vi "read_stimulus_h5.vi"(11 "Path":path) -> (0 "error out":errorcluster, 3 "output cluster":T1, 4 "alignment_command":i32[](array[numeric]), 6 "piezo_command":i32[](array[numeric]))   [LabVIEW 2015]
uses:
  <vilib>/addons/h5labview2/file/H5Fmode.ctl
  <vilib>/addons/h5labview2/base/lib_path.vi
  <vilib>/addons/h5labview2/base/H5Equery.vi
  <vilib>/addons/h5labview2/base/hid_t.ctl
  <vilib>/addons/h5labview2/dataset/H5Dread.llb/H5Dread.xnode
  <vilib>/addons/h5labview2/file/H5F.lvlib
  <vilib>/addons/h5labview2/group/H5G.lvlib
panel:
  out "Alignment Command":dbl[](graph)
  out "Piezo Command":dbl[](graph)
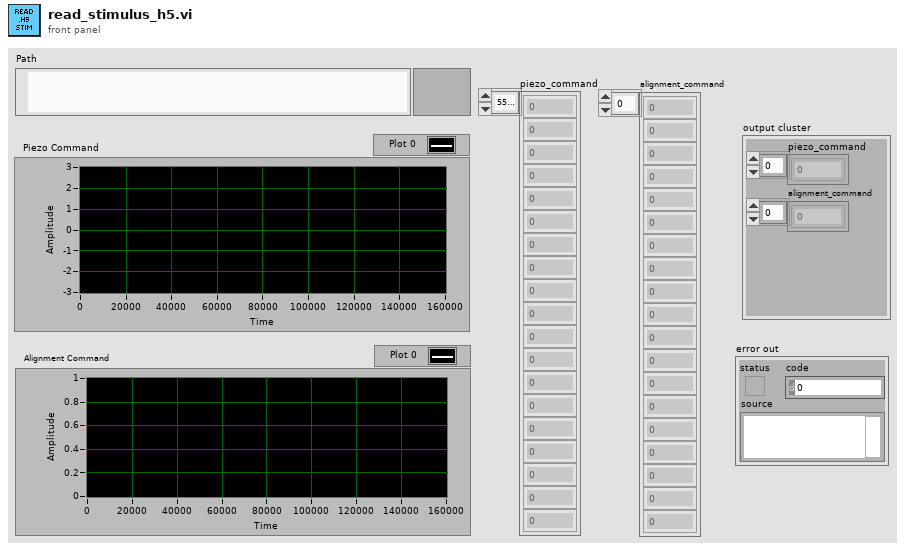
[diagram p1: front panel]
types:
  T1 = cluster{"piezo_command":dbl[], "alignment_command":dbl[]}
  T2 = typedef "H5F.lvlib/H5Fmode.ctl" = enum16{"read-only", "read-write", "overwrite", "create new", "open or create"}
  T3 = typedef "hid_t.ctl" = i32
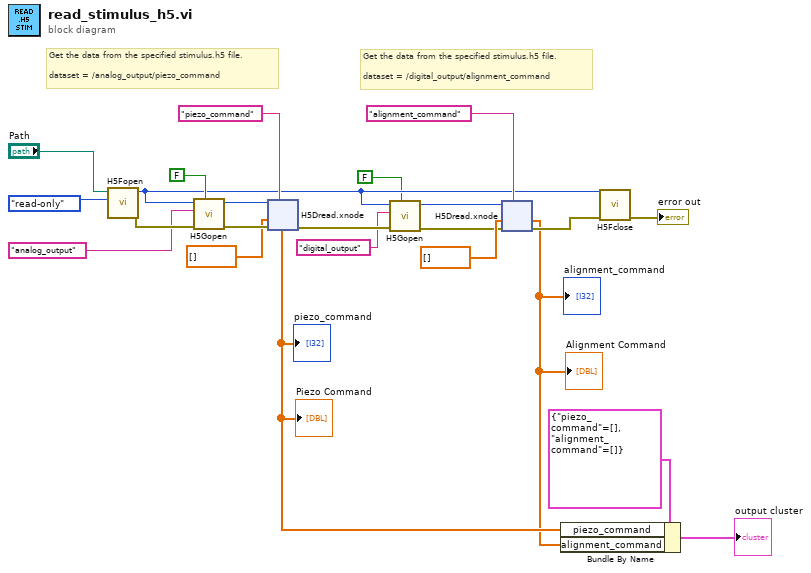
[diagram p0: block diagram]
diagram:
  # "Get the data from the specified stimulus.h5 file.\n\ndataset = /analog_output/piezo_command"
  # "Get the data from the specified stimulus.h5 file.\n\ndataset = /digital_output/alignment_command"
  n1 = call <vilib>:"H5Fopen.vi"("mode (read-only)"=H5Fmode."read-only" ("mode"), "path"="Path") -> ("error out"=w22:errorcluster, "ref out"=w3:T3)  [unwired: 8 in]
  n2 = call <vilib>:"H5Gopen.vi"("create? (F)"=FALSE, "error in (no error)"=w22, "name"="analog_output", "ref in"=w3) -> ("error out"=w20:errorcluster, "group out"=w16:T3)  [unwired: 6 in]
  n3 = xnode "H5Dread.xnode"("dataset name (this)"="piezo_command" ("name"), "error in (no error)"=w20, "default"=dbl[] [] ("data"), "ref in"=w16) -> ("error out"=w6:errorcluster, "data"=w9:dbl[])  [unwired: 2 in, 2 out]
  "piezo_command" <- w9
  "Piezo Command" <- w9
  n4 = call <vilib>:"H5Gopen.vi"("create? (F)"=FALSE, "error in (no error)"=w6, "name"="digital_output", "ref in"=w3) -> ("error out"=w5:errorcluster, "group out"=w4:T3)  [unwired: 6 in]
  n5 = xnode "H5Dread.xnode"("dataset name (this)"="alignment_command" ("name"), "error in (no error)"=w5, "default"=dbl[] [] ("data"), "ref in"=w4) -> ("error out"=w11:errorcluster, "data"=w8:dbl[])  [unwired: 2 in, 2 out]
  "alignment_command" <- w8
  "Alignment Command" <- w8
  n6 = Bundle By Name(cluster=T1 {"piezo_command"=[], "alignment_command"=[]}, "piezo_command"=w9, "alignment_command"=w8) -> (→"output cluster":T1)
  n7 = call <vilib>:"H5Fclose.vi"("error in (no error)"=w11, "ref"=w3) -> ("error out"=→"error out":errorcluster)  [unwired: 9 in]
